vi "core_code_mod_toolbox.vi"(2 "error code":i32) -> (7 "local code":i32, 9 "toolbox offset":i32)   [LabVIEW 2015]
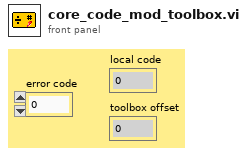
[diagram p1: front panel]
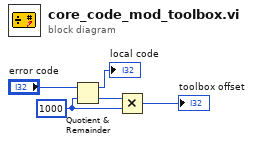
[diagram p0: block diagram]
diagram:
  w2 = 1000 ("y")
  n1 = Quotient & Remainder(x="error code", y=w2) -> (x-y*floor(x/y)=→"local code":i32, floor(x/y)=w3:i32)
  n2 = Multiply(x=w3, y=w2) -> (x*y=→"toolbox offset":i32)
